vi "Pre Launch Init.vi"(11 "Nested in":refnum<class "Logger Normal.lvclass">) -> (0 "error out":errorcluster, 3 "Nested out":refnum<class "Logger Normal.lvclass">)   [LabVIEW 2020, in "Logger Normal.lvlib" / "Logger Normal.lvclass"]
doc: "(<B>Filename</B>: Actor Framework.lvlib:Actor.lvclass:Pre Launch Init.vi)\n\nDefines behavior that occurs after the Launch Nested Actor method is invoked but before the actor's Actor Core method begins running.\n\nBy default, this method does nothing. A descendant class may override it to define behavior."
uses:
  Logger Normal.lvclass
  Logger/Logger/Logger.lvclass
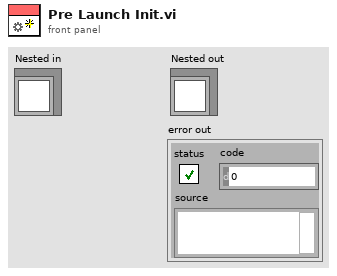
[diagram p1: front panel]
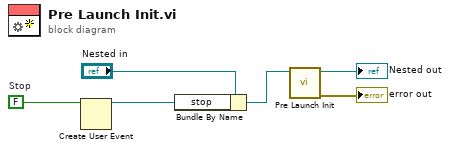
[diagram p0: block diagram]
diagram:
  w5 = FALSE  # Stop
  n1 = Create User Event(user event datatype=w5) -> (user event=w4:refnum<user-event>)  [unwired: 1 in, 1 out]
  n2 = Bundle By Name ("Bundle Events")(cluster="Nested in", "stop"=w4) -> (w3:refnum<class "Logger Normal.lvclass">)
  n3 = call-parent "Pre Launch Init.vi"("Actor in"=w3) -> ("error out"=→"error out":errorcluster, "Actor out"=→"Nested out":refnum<class "Logger Normal.lvclass">)  [unwired: 9 in]
